vi "简易温度转换器.vi"() -> ()   [LabVIEW 2012, in "Temp Converter.lvlib"]
uses:
  Temp Converter.lvlib
  FtoC/F to C (dbl).vi
  CtoF/C to F (dbl).vi
  KtoC/K to C (dbl).vi
  CtoK/C to K (dbl).vi
  KtoF/K to F(dbl).vi
  FtoK/F to K(dbl).vi
panel:
  in  "停止":bool
  in  "转换模式":T1(ring)
  out "转换温度":dbl(slide) scale=-300.0..300.0
  in  "输入温度":dbl(slide) scale=-300.0..300.0
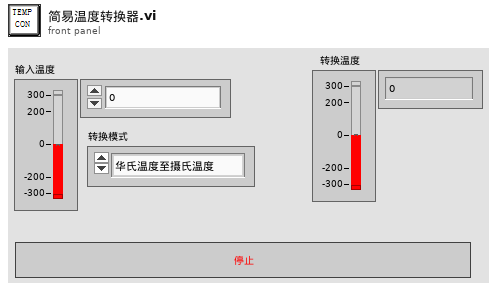
[diagram p1: front panel]
types:
  T1 = enum16{"华氏温度至摄氏温度", "摄氏温度至华氏温度", "开氏温度至摄氏温度", "摄氏温度至开氏温度", "开氏温度至华氏温度", "华氏温度至开氏温度"}
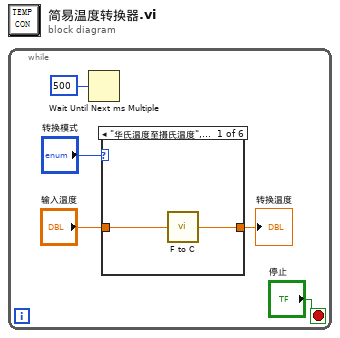
[diagram p0: block diagram]
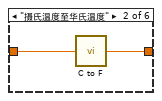
[diagram p2: hidden frame]
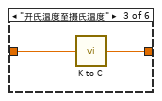
[diagram p3: hidden frame]
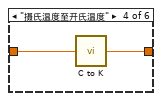
[diagram p4: hidden frame]
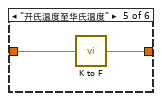
[diagram p5: hidden frame]
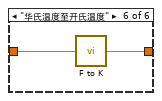
[diagram p6: hidden frame]
diagram:
  n1 = while {
    stop <- "停止" stop-if-true
    n2 = Wait Until Next ms Multiple(millisecond multiple=u32 500 ("毫秒倍数")) -> ()  [unwired: 1 out]
    n3 = case shown="\"华氏温度至摄氏温度\", 默认" "转换模式" {
      tunnel: "输入温度" -> [w7 w9 w11 w13 w15 w17]
      tunnel: [w6 w8 w10 w12 w14 w16] -> w1
      frame "华氏温度至摄氏温度", Default {
        n4 = call-poly "F to C.vi"("F"=w7) -> ("C"=w6:dbl)
      }
      frame "摄氏温度至华氏温度" {
        n5 = call-poly "C to F.vi"("C"=w9) -> ("F"=w8:dbl)
      }
      frame "开氏温度至摄氏温度" {
        n6 = call-poly "K to C.vi"("K"=w11) -> ("C"=w10:dbl)
      }
      frame "摄氏温度至开氏温度" {
        n7 = call-poly "C to K.vi"("C"=w13) -> ("K"=w12:dbl)
      }
      frame "开氏温度至华氏温度" {
        n8 = call-poly "K to F.vi"("K"=w15) -> ("F"=w14:dbl)
      }
      frame "华氏温度至开氏温度" {
        n9 = call-poly "F to K.vi"("F"=w17) -> ("K"=w16:dbl)
      }
    }
    "转换温度" <- w1
  }
